vi "check sr.vi"(7 "file path (use dialog)":path=path "D:/Configuration Folder Barcode/srno", 9 "sr. no":i32, 11 "writeL:t":bool) -> (0 "sr. out":i32)   [LabVIEW 2024]
panel:
  out "error out":errorcluster
  out "appended path":path
  out "date/time string 2":string
  out "date/time string":string
  out "read":cluster{"date":timestamp, "sr. no":i32}
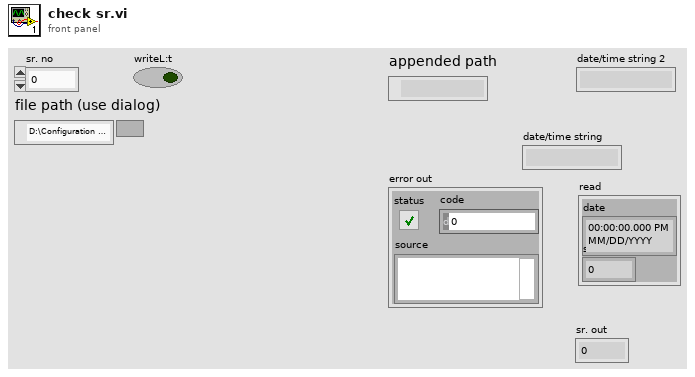
[diagram p1: front panel]
types:
  T1 = enum16{"open", "replace", "create", "open or create", "replace or create", "replace or create with confirmation"}
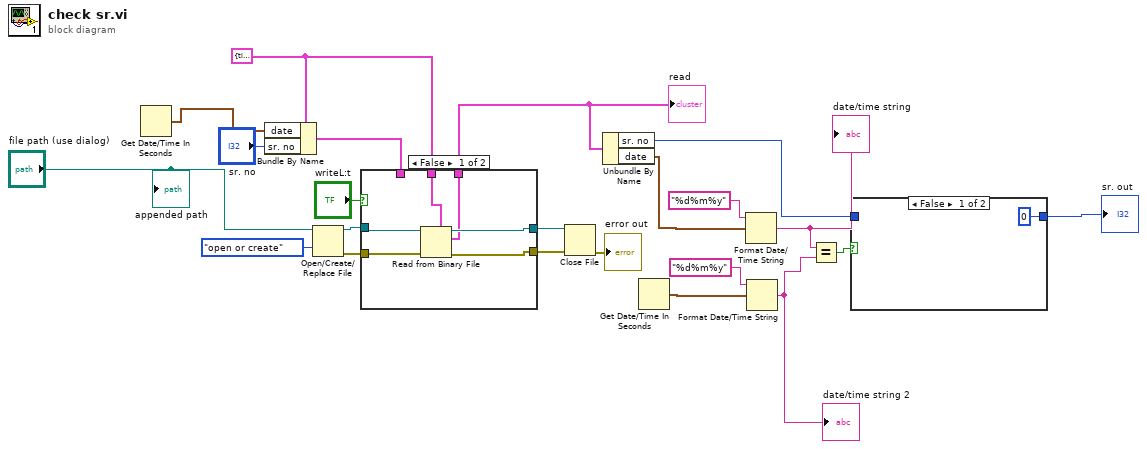
[diagram p0: block diagram]
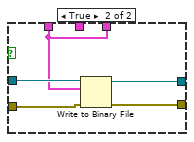
[diagram p3: hidden frame]
diagram:
  w6 = cluster{"date":timestamp, "sr. no":i32} {"date"=timestamp(0 s since 1904-01-01), "sr. no"=0} ("read")
  n1 = Get Date/Time In Seconds() -> (seconds since 1Jan1904=w5:timestamp)
  n2 = Bundle By Name(cluster=w6, "date"=w5, "sr. no"="sr. no") -> (w3:cluster{"date":timestamp, "sr. no":i32})
  n3 = Open/Create/Replace File(file path (use dialog)="file path (use dialog)", operation (0:open)=T1."open or create") -> (refnum out=w22:refnum<file>, error out=w21:errorcluster)  [unwired: 4 in, 1 out]
  n4 = case shown="False" "writeL:t" {
    tunnel: w22 -> [w28 w33]
    tunnel: w21 -> [w27 w32]
    tunnel: [w26 w31] -> w20
    tunnel: [w25 w30] -> w19
    tunnel: w6 -> [w24 _]
    tunnel: [w23 w29] -> w16
    tunnel: w3 -> [_ w29]
    frame False {
      n5 = Read from Binary File(5:w24, 8:w27, 11:w28) -> (0:w26:errorcluster, 2:w23:cluster{"date":timestamp, "sr. no":i32}, 3:w25:refnum<file>)  [unwired: 3 in, 1 out]
    }
    frame True {
      n6 = Write to Binary File(file (use dialog)=w33, data=w29, error in=w32) -> (refnum out=w30:refnum<file>, error out=w31:errorcluster)  [unwired: 3 in, 1 out]
    }
  }
  "read" <- w16
  n7 = Close File(refnum=w19, error in=w20) -> (error out=→"error out":errorcluster)  [unwired: 1 out]
  n8 = Unbundle By Name(w16) -> ("sr. no"=w8:i32, "date"=w13:timestamp)
  n9 = Get Date/Time In Seconds() -> (seconds since 1Jan1904=w15:timestamp)
  n10 = Format Date/Time String(time format string (%c)="%d%m%y", seconds (now)=w13) -> (date/time string=w11:string)  [unwired: 1 in]
  "date/time string" <- w11
  n11 = Format Date/Time String(time format string (%c)="%d%m%y", seconds (now)=w15) -> (date/time string=w10:string)  [unwired: 1 in]
  "date/time string 2" <- w10
  n12 = Equal?(x=w11, y=w10) -> (x = y?=w9:bool)
  n13 = case shown="False" w9 {
    tunnel: w8 -> [_ w35]
    tunnel: [0 ("sr. no") w35] -> w7
    frame False {
    }
    frame True {
    }
  }
  "sr. out" <- w7
  "appended path" <- "file path (use dialog)"
